vi "ADIS16470 Initialize DMA Odometry.vi"(6 "Encoder R":T1={"DevStatus"={"status"=FALSE, "code"=0, "source"=""}, "EncoderIndex"=enum."Invalid", "CounterIndex"=enum."Invalid", "DistancePerCount"=1.0, "Decoding Type"=enum."4x"}, 7 "Encoder L":T1={"DevStatus"={"status"=FALSE, "code"=0, "source"=""}, "EncoderIndex"=enum."Invalid", "CounterIndex"=enum."Invalid", "DistancePerCount"=1.0, "Decoding Type"=enum."4x"}, 8 "error in":errorcluster, 9 "Calibration Time":T5, 11 "ADIS16470DevRef":T7={"DevStatus"={"status"=FALSE, "code"=0, "source"=""}, "Hardware Config"={"SPI Clock Rate (Hz)"=1000000.0, "IMU SPI Mode (3)"=enum."Mode 3 (Clk Idle High,Sample on Trailing)", "IMU Reset Pin"=enum."SPI Port CS2", "IMU SPI Bus"=enum."SPI On-Board, CS0", "IMU Data Ready Pin"=enum."SPI Port CS1", "Stall Config"={"Pow2BytesPerRead"=255, "StallTicks"=640, "CsToSclkTicks"=5}}, "Calibration Complete"=refnum, "Status FIFO"=refnum, "Last Value Reference"=refnum, "Sychronous Process VI"=refnum, "Cmd FIFO"=refnum, "Source"={"DevStatus"={"status"=FALSE, "code"=0, "source"=""}, "AnalogTriggerMode?"=FALSE, "DigitalMode"={"DIO Channel"=enum."Disabled"}, "AnalogTriggerMode"={"AnalogTriggerIndex"=enum."Trig 0", "OutputType"=enum."InWindow"}}, "Data FIFO"=refnum, "Calibration Time"=enum."1s"}) -> (0 "error out":errorcluster)   [LabVIEW 2019]
uses:
  Typedef/ADIS16470 Device Reference.ctl
  Typedef/ADIS16470 Hardware Configuration.ctl
  <vilib>/Rock Robotics/WPI/SPI/WPI_SPIMode.ctl
  <vilib>/Rock Robotics/SystemInterfaces/DIO/FPGA_DIOChannel.ctl
  <vilib>/Rock Robotics/SystemInterfaces/spilib/spi_bus.ctl
  Typedef/ADIS16470 Status.ctl
  Typedef/ADIS16470 Data.ctl
  Typedef/ADIS16470 Process.ctl
  Typedef/ADIS16470 Command Type.ctl
  <vilib>/Rock Robotics/SystemInterfaces/CounterEncoderSourceConvertion/FPGA_CounterEncoderSourceConvertionLVSourceType.ctl
  <vilib>/Rock Robotics/SystemInterfaces/DIO/FPGA_DIODigitalSourceChannel.ctl
  <vilib>/Rock Robotics/SystemInterfaces/AnalogTrigger/FPGA_AnalogTriggerIndex.ctl
  <vilib>/Rock Robotics/SystemInterfaces/AnalogTrigger/FPGA_AnalogTriggerOutType.ctl
  Typedef/ADIS16470 Calibration Time.ctl
  <vilib>/Rock Robotics/WPI/Encoder/WPI_EncoderDevRef.ctl
  <vilib>/Rock Robotics/SystemInterfaces/Encoder/FPGA_EncoderIdx.ctl
  <vilib>/Rock Robotics/SystemInterfaces/Counter/FPGA_CounterCtrSystemIndex.ctl
  <vilib>/Rock Robotics/WPI/Encoder/WPI_EncoderType.ctl
  <vilib>/Rock Robotics/WPI/SPI/WPI_SPIDevRef.ctl
  Typedef/ADIS16470 Register.ctl
  <vilib>/Rock Robotics/WPI/DMA/WPI_DMARef.ctl
  Typedef/ADIS16470 State Machine.ctl
  <vilib>/Rock Robotics/WPI/DMA/WPI_DMAEncoderOutputType.ctl
  Support Code/Indicator LED - Green.ctl
  Support Code/Indicator LED Indexes.ctl
  <vilib>/Rock Robotics/WPI/Counter/WPI_CounterDigitalInputToDigitalSource.vi
  <vilib>/Rock Robotics/WPI/DMA/WPI_DMAOpenExternal.vi
  <vilib>/Rock Robotics/WPI/DMA/WPI_DMAAddChannelToStream_Encoder.vi
  <vilib>/Rock Robotics/WPI/DMA/WPI_DMAAddChannelToStream_Timestamp.vi
panel:
  out "Array2Prev":u32[](array[numeric])
  out "ArrayPrev":u32[](array[numeric])
  out "Array 2":u32[](array[numeric])
  out "Array":u32[](array[numeric])
  in  "element":T6
  out "Waveform Chart":dbl(graph)
  out "Offset Bias":i16[](array[numeric])
  # "XG_BIAS_LOW"
  # "XG_BIAS_HIGH"
  # "YG_BIAS_LOW"
  # "YG_BIAS_HIGH"
  # "ZG_BIAS_LOW"
  # "ZG_BIAS_HIGH"
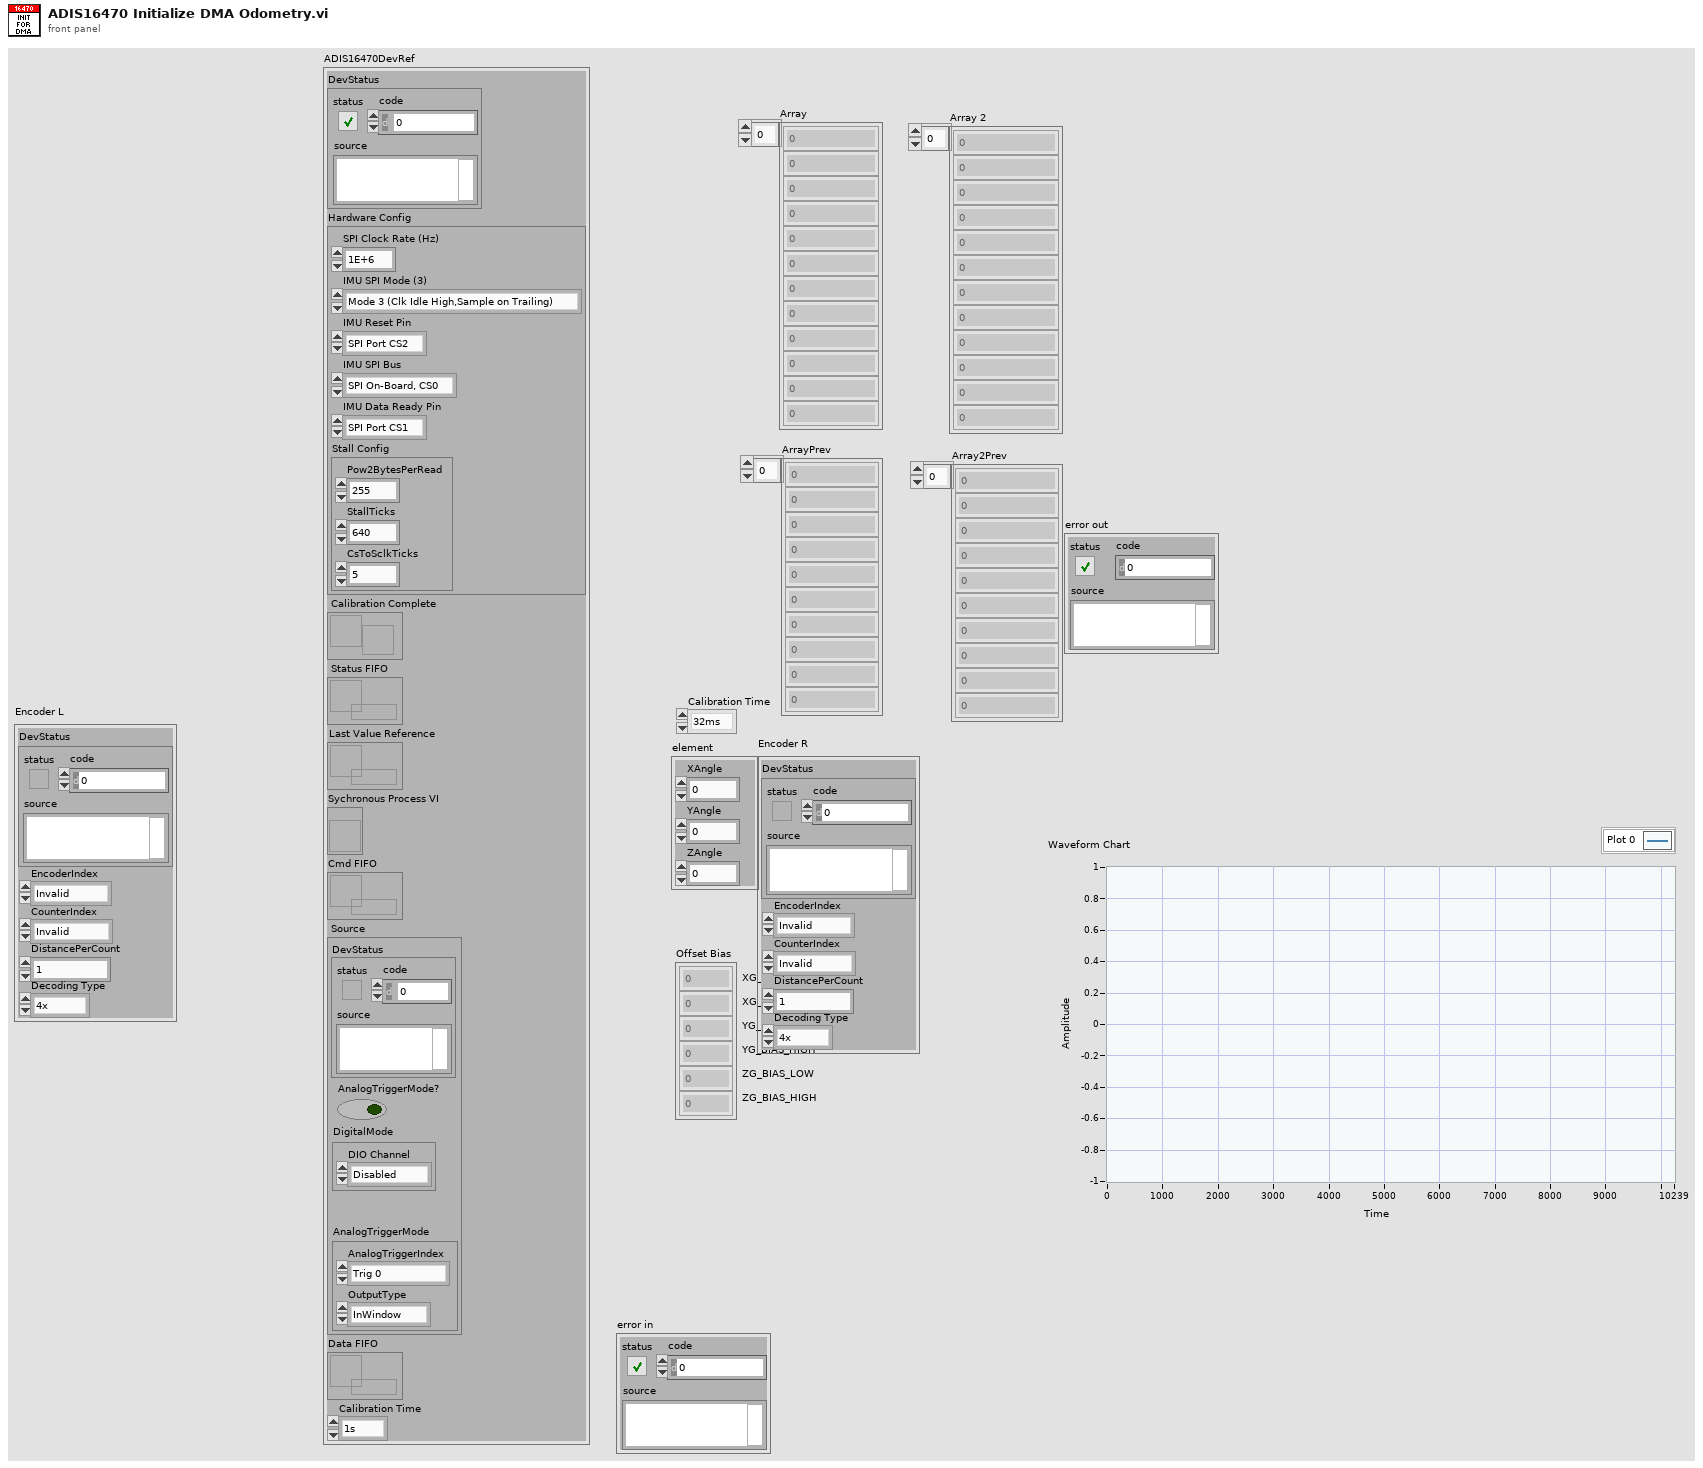
[diagram p1: front panel]
types:
  T1 = typedef "WPI_EncoderDevRef.ctl" = cluster{"DevStatus":errorcluster, "EncoderIndex":T2, "CounterIndex":T3, "DistancePerCount":dbl, "Decoding Type":T4}
  T2 = typedef "FPGA_EncoderIdx.ctl" = enum8{"Enc 0", "Enc 1", "Enc 2", "Enc 3", "Enc 4", "Enc 5", "Enc 6", "Enc 7", "Invalid"}
  T3 = typedef "FPGA_CounterCtrSystemIndex.ctl" = enum8{"Ctr 0", "Ctr 1", "Ctr 2", "Ctr 3", "Ctr 4", "Ctr 5", "Ctr 6", "Ctr 7", "Invalid"}
  T4 = typedef "WPI_EncoderType.ctl" = enum16{"1x", "2x", "4x"}
  T5 = typedef "ADIS16470 Calibration Time.ctl" = enum16{"32ms", "64ms", "128ms", "256ms", "512ms", "1s", "2s", "4s", "8s", "16s", "32s", "64s"}
  T6 = typedef "ADIS16470 Data.ctl" = cluster{"XAngle":dbl, "YAngle":dbl, "ZAngle":dbl}
  T7 = typedef "ADIS16470 Device Reference.ctl" = cluster{"DevStatus":errorcluster, "Hardware Config":T8, "Calibration Complete":refnum<notifier>, "Status FIFO":refnum<k33>, "Last Value Reference":refnum<data-value>, "Sychronous Process VI":T12, "Cmd FIFO":refnum<k33>, "Source":T13, "Data FIFO":refnum<k33>, "Calibration Time":T5}
  T8 = typedef "ADIS16470 Hardware Configuration.ctl" = cluster{"SPI Clock Rate (Hz)":dbl, "IMU SPI Mode (3)":T9, "IMU Reset Pin":T10, "IMU SPI Bus":T11, "IMU Data Ready Pin":T10, "Stall Config":cluster{"Pow2BytesPerRead":u8, "StallTicks":u16, "CsToSclkTicks":u8}}
  T9 = typedef "WPI_SPIMode.ctl" = enum16{"Mode 0 (Clk Idle Low,Sample on Leading)", "Mode 1 (Clk Idle Low,Sample on Trailing)", "Mode 2 (Clk Idle High,Sample on Leading)", "Mode 3 (Clk Idle High,Sample on Trailing)"}
  T10 = typedef "FPGA_DIOChannel.ctl" = enum8{"DIO 0", "DIO 1", "DIO 2", "DIO 3", "DIO 4", "DIO 5", "DIO 6", "DIO 7", "DIO 8", "DIO 9", "DIO MXP 0", "DIO MXP 1", "DIO MXP 2", "DIO MXP 3", "DIO MXP 4", "DIO MXP 5", "DIO MXP 6", "DIO MXP 7", "DIO MXP 8", "DIO MXP 9", "DIO MXP 10", "DIO MXP 11", "DIO MXP 12", "DIO MXP 13", "DIO MXP 14", "DIO MXP 15", "SPI Port CS1", "SPI Port CS2", "SPI Port CS3", "SPI Port MISO", "SPI Port MOSI", "Invalid"}
  T11 = typedef "spi_bus.ctl" = enum16{"SPI On-Board, CS0", "SPI On-Board, CS1", "SPI On-Board, CS2", "SPI On-Board, CS3", "SPI MXP", "Invalid"}
  T12 = typedef "ADIS16470 Process.ctl" = refnum<vi>
  T13 = typedef "FPGA_CounterEncoderSourceConvertionLVSourceType.ctl" = cluster{"DevStatus":errorcluster, "AnalogTriggerMode?":bool, "DigitalMode":cluster{"DIO Channel":T14}, "AnalogTriggerMode":cluster{"AnalogTriggerIndex":T15, "OutputType":T16}}
  T14 = typedef "FPGA_DIODigitalSourceChannel.ctl" = enum8{"DIO 0", "DIO 1", "DIO 2", "DIO 3", "DIO 4", "DIO 5", "DIO 6", "DIO 7", "DIO 8", "DIO 9", "DIO MXP 0", "DIO MXP 1", "DIO MXP 2", "DIO MXP 3", "DIO MXP 4", "DIO MXP 5", "DIO MXP 6", "DIO MXP 7", "DIO MXP 8", "DIO MXP 9", "DIO MXP 10", "DIO MXP 11", "DIO MXP 12", "DIO MXP 13", "DIO MXP 14", "DIO MXP 15", "SPI Port CS1", "SPI Port CS2", "SPI Port CS3", "SPI Port MISO", "SPI Port MOSI", "Disabled"}
  T15 = typedef "FPGA_AnalogTriggerIndex.ctl" = enum8{"Trig 0", "Trig 1", "Trig 2", "Trig 3", "Trig 4", "Trig 5", "Trig 6", "Trig 7", "Invalid"}
  T16 = typedef "FPGA_AnalogTriggerOutType.ctl" = enum16{"InWindow", "TriggerState", "Rising", "Falling"}
  T17 = typedef "ADIS16470 State Machine.ctl" = enum16{"Error", "Reset", "Register DR Source", "Start SPI", "Write Config", "Calibrate", "Write Run Config", "Init Encoder DMA", "Init Auto SPI", "Decode AutoSPI", "Decode Encoder DMA", "Process", "Run Cmds", "Close"}
  T18 = typedef "WPI_SPIDevRef.ctl" = cluster{"DevStatus":errorcluster, "Handle":i32, "SPI Bus":T11}
  T19 = typedef "ADIS16470 Register.ctl" = u8
  T20 = typedef "WPI_DMARef.ctl" = cluster{"DevStatus":errorcluster, "Host Buffer Depth (Samples)":u32}
  T21 = cluster{"SPIDevRef":T18, "Data Counter":u16, "Reset":bool, "Data Ready Source":T13, "Bytes Per Sample":u32, "Data":dbl[], "ADIS16470DevRef":T7, "TimeStampPrev":u32, "Sensor to Robot Rotation":dbl[][], "Data Packet":T19[], "AutoSPI Active?":bool, "Encoder L":T1, "Encoder R":T1, "DMARef":T20, "IMU Raw":cluster{"Theta":dbl[], "Timestamp":u32}[], "Encoder Raw":cluster{"Encoder R":u32, "Encoder L":u32, "Timestamp":u32}[]}
  T22 = typedef "ADIS16470 Status.ctl" = cluster{"Calibrated?":bool, "IMU Detected?":bool}
  T23 = cluster{"DigitalSource":T13, "Edge":enum16{"Rising Edge", "Falling Edge", "Raising & Falling Edge", "Disabled"}}
  T24 = typedef "Indicator LED Indexes.ctl" = enum16{"Code Started", "DS Connected", "Limelight", "Turret Calibrated", "Gyro Calibrated", "USB0 Connected", "USB1 Connected", "FMS Attached"}
  T25 = typedef "Indicator LED - Green.ctl" = u32
  T26 = typedef "ADIS16470 Command Type.ctl" = cluster{"Command":enum16{"None", "Reset", "Set Calibration Period", "Recalibrate", "Recal Complete", "Exit Auto SPI", "Start Auto SPI"}, "Data":u32}
  T27 = typedef "WPI_DigitalOutputDevRef.ctl" = cluster{"DIO Channel":T10, "DevStatus":errorcluster}
  T28 = typedef "WPI_DigitalInputDevRef.ctl" = cluster{"DevStatus":errorcluster, "DIO Channel":T10}
  T29 = typedef "WPI_DMAEncoderOutputType.ctl" = enum16{"Encoder Value", "Timer Value"}
  T30 = cluster{"DigitalSource":T13, "Edge":enum16{"Rising Edge", "Falling Edge", "Raising & Falling Edge", "Disabled"}}[]
  T31 = cluster{"Pow2BytesPerRead":u8, "StallTicks":u16, "CsToSclkTicks":u8}
  T32 = cluster{"Encoder R":i32, "Encoder L":i32, "Timestamp":u32}[]
  T33 = cluster{"Encoder R":u32, "Encoder L":u32, "Timestamp":u32}[]
  T34 = enum16{"None", "Reset", "Set Calibration Period", "Recalibrate", "Recal Complete", "Exit Auto SPI", "Start Auto SPI"}
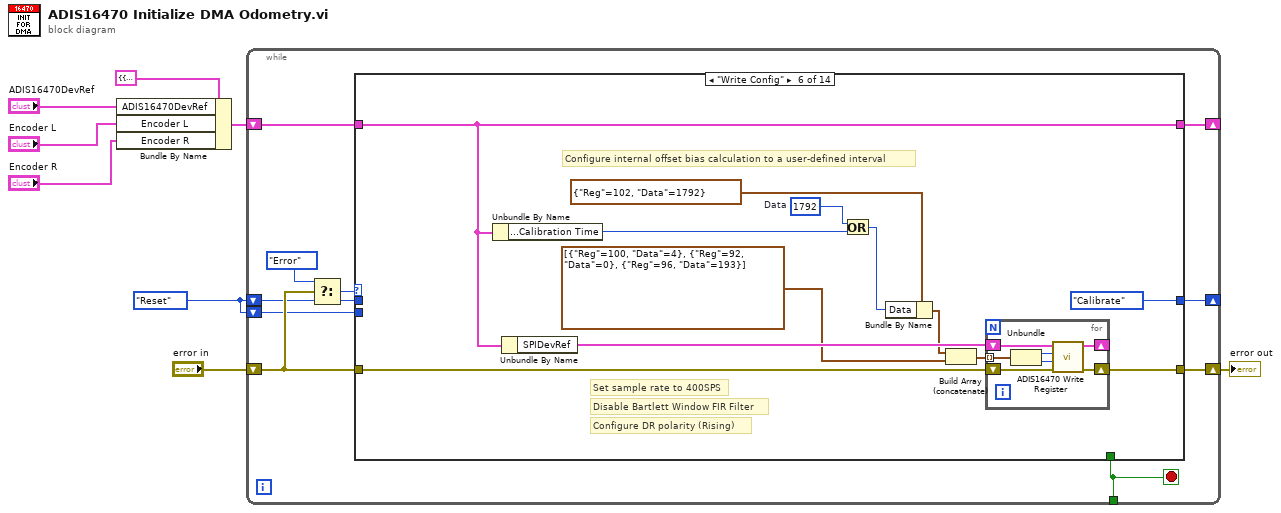
[diagram p0: block diagram]
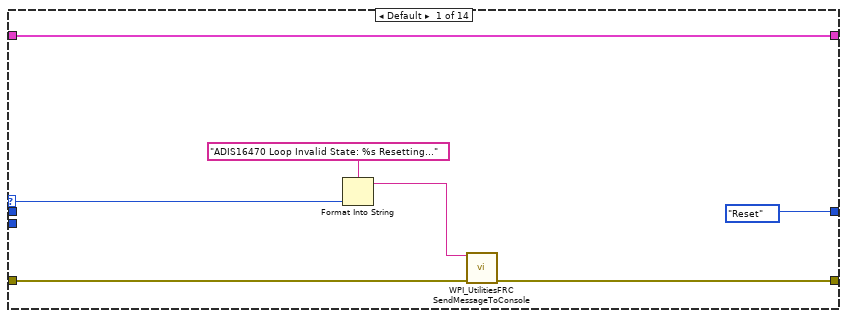
[diagram p2: hidden frame]
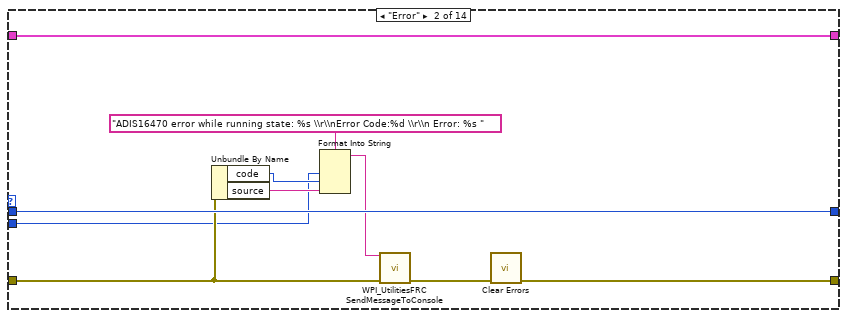
[diagram p3: hidden frame]
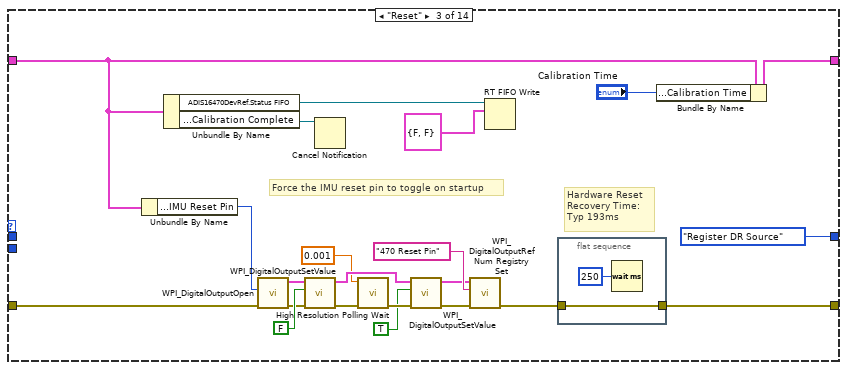
[diagram p4: hidden frame]
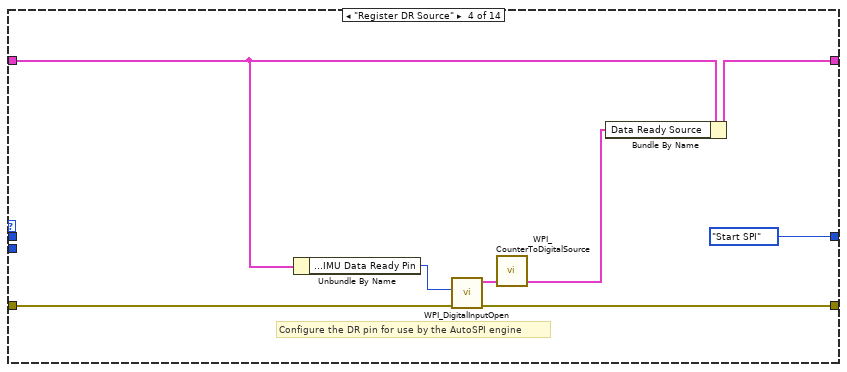
[diagram p5: hidden frame]
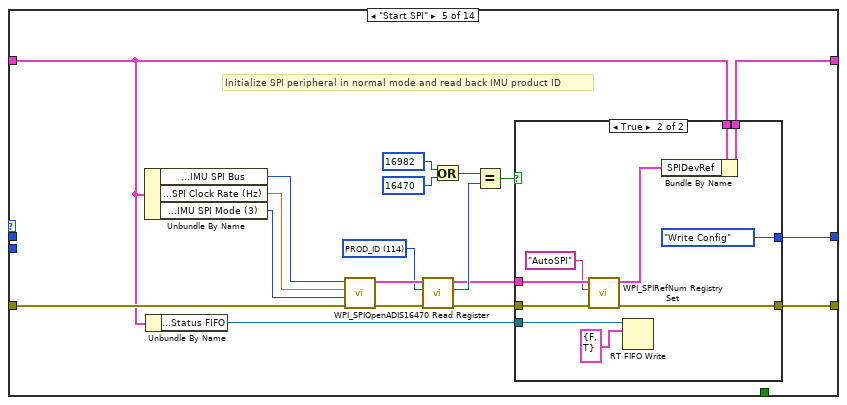
[diagram p6: hidden frame]
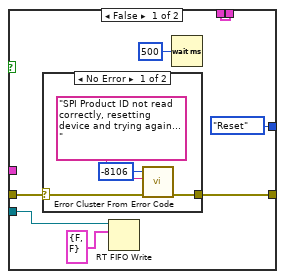
[diagram p7: hidden frame]
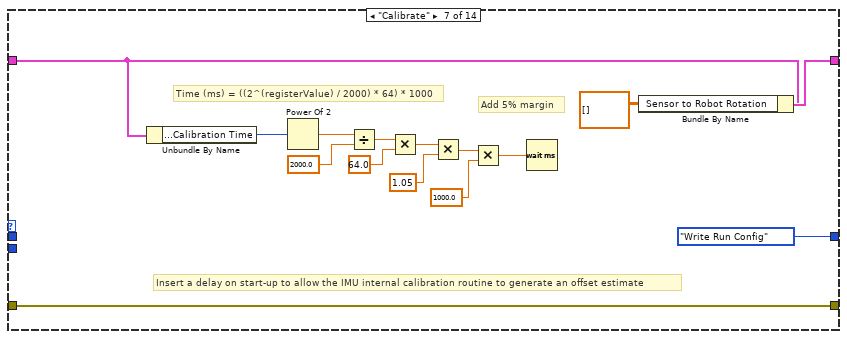
[diagram p9: hidden frame]
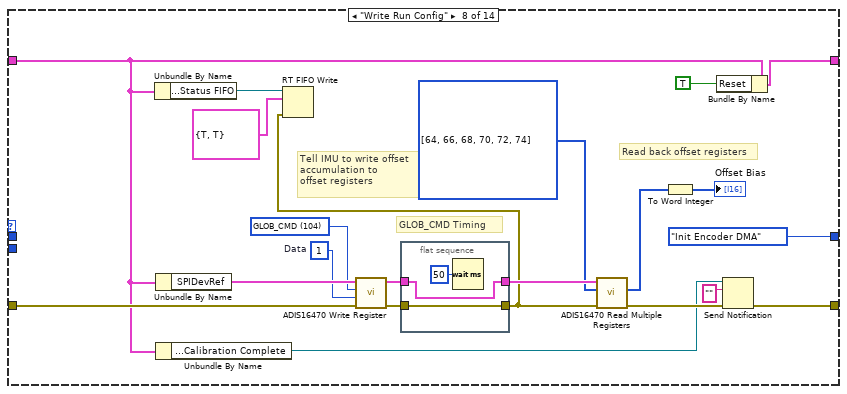
[diagram p10: hidden frame]
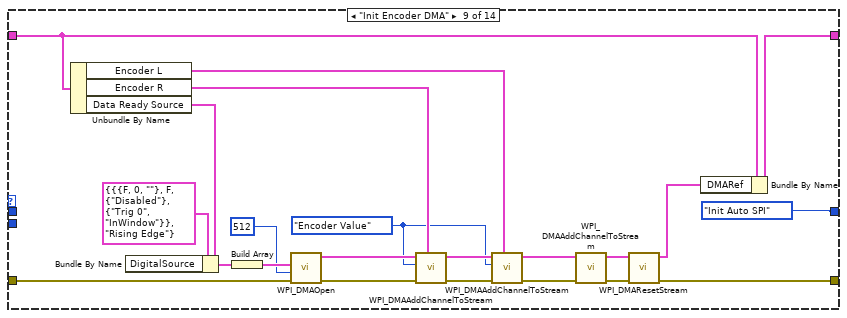
[diagram p11: hidden frame]
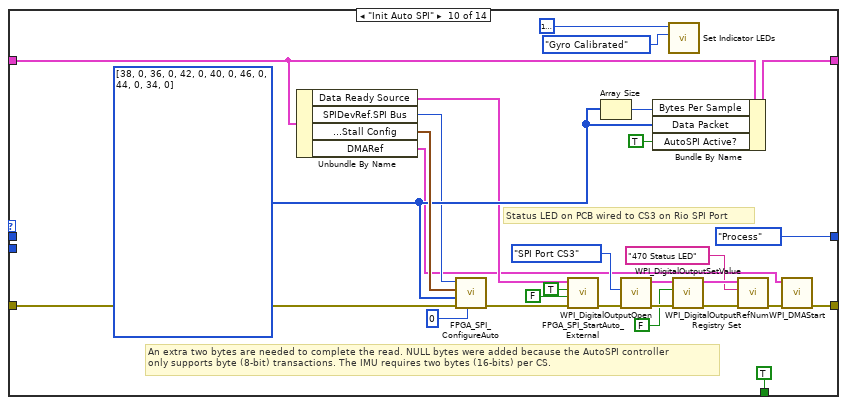
[diagram p12: hidden frame]
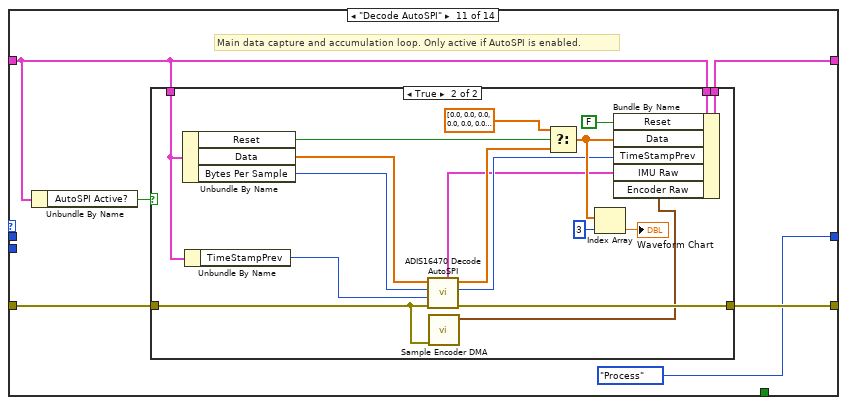
[diagram p13: hidden frame]
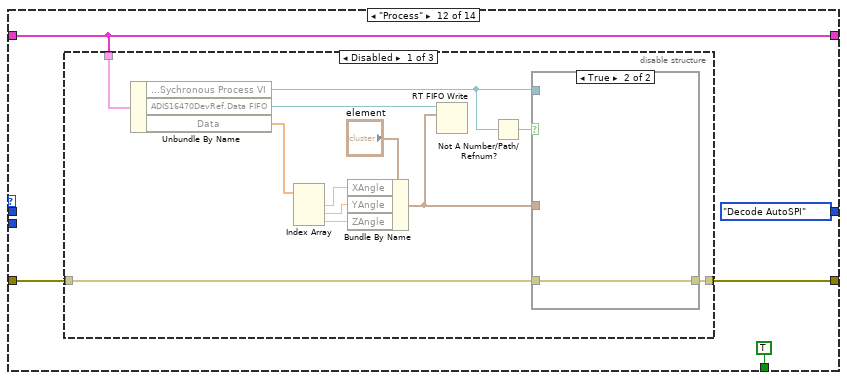
[diagram p15: hidden frame]
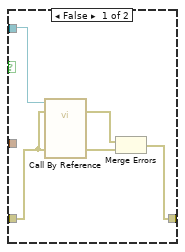
[diagram p16: hidden frame]
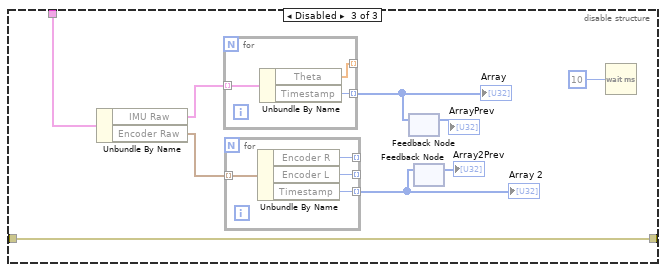
[diagram p18: hidden frame]
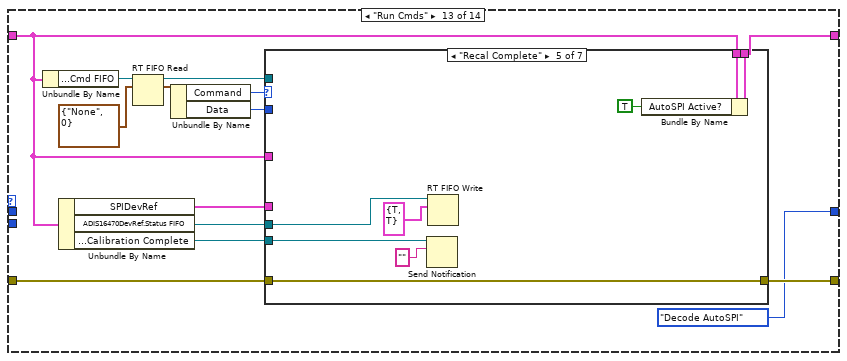
[diagram p19: hidden frame]
diagram:
  w4 = ADIS16470_State_Machine."Reset" ("ADIS16470 State Machine")
  n1 = Bundle By Name(cluster=T21 {"SPIDevRef"={"DevStatus"={"status"=FALSE, "code"=0, "source"=""}, "Handle"=0, "SPI Bus"=enum."SPI On-Board, CS0"}, "Data Counter"=0, "Reset"=FALSE, "Data Ready Source"={"DevStatus"={"status"=FALSE, "code"=0, "source"=""}, "AnalogTriggerMode?"=FALSE, "DigitalMode"={"DIO Channel"=enum."DIO 1"}, "AnalogTriggerMode"={"AnalogTriggerIndex"=enum."Trig 0", "OutputType"=enum."InWindow"}}, "Bytes Per Sample"=0, "Data"=[0.0, 0.0, 0.0, 0.0, 0.0, 0.0, 0.0, 0.0], "ADIS16470DevRef"={"DevStatus"={"status"=FALSE, "code"=0, "source"=""}, "Hardware Config"={"SPI Clock Rate (Hz)"=1000000.0, "IMU SPI Mode (3)"=enum."Mode 3 (Clk Idle High,Sample on Trailing)", "IMU Reset Pin"=enum."SPI Port CS2", "IMU SPI Bus"=enum."SPI On-Board, CS0", "IMU Data Ready Pin"=enum."SPI Port CS1", "Stall Config"={"Pow2BytesPerRead"=255, "StallTicks"=640, "CsToSclkTicks"=5}}, "Calibration Complete"=refnum, "Status FIFO"=refnum, "Last Value Reference"=refnum, "Sychronous Process VI"=refnum, "Cmd FIFO"=refnum, "Source"={"DevStatus"={"status"=FALSE, "code"=0, "source"=""}, "AnalogTriggerMode?"=FALSE, "DigitalMode"={"DIO Channel"=enum."Disabled"}, "AnalogTriggerMode"={"AnalogTriggerIndex"=enum."Trig 0", "OutputType"=enum."InWindow"}}, "Data FIFO"=refnum, "Calibration Time"=enum."1s"}, "TimeStampPrev"=0, "Sensor to Robot Rotation"=[], "Data Packet"=[38, 0, 36, 0, 42, 0, 40, 0, 46, 0, 44, 0, 114, 0], "AutoSPI Active?"=TRUE, "Encoder L"={"DevStatus"={"status"=FALSE, "code"=0, "source"=""}, "EncoderIndex"=enum."Invalid", "CounterIndex"=enum."Invalid", "DistancePerCount"=1.0, "Decoding Type"=enum."4x"}, "Encoder R"={"DevStatus"={"status"=FALSE, "code"=0, "source"=""}, "EncoderIndex"=enum."Invalid", "CounterIndex"=enum."Invalid", "DistancePerCount"=1.0, "Decoding Type"=enum."4x"}, "DMARef"={"DevStatus"={"status"=FALSE, "code"=0, "source"=""}, "Host Buffer Depth (Samples)"=0}, "IMU Raw"=[], "Encoder Raw"=[]}, "ADIS16470DevRef"="ADIS16470DevRef", "Encoder L"="Encoder L", "Encoder R"="Encoder R") -> (w7:T21)
  n2 = while {
    shift-right: [w15] -> _
    shift-left: w4 -> [w12]
    shift-right: [w17] -> _
    shift-left: w7 -> [w18]
    shift-right: [w16] -> w1
    shift-left: "error in" -> [w14]
    shift-left: w4 -> [w11]
    tunnel: [w9] -> _
    stop <- w9 stop-if-true
    n3 = Select(t=ADIS16470_State_Machine."Error" ("ADIS16470 State Machine"), s=w14, f=w12) -> (s? t:f=w13:T17)
    n4 = case shown="\"Write Config\"" w13 {
      selector: w13 -> [w24 _ _ _ _ _ _ _ _ _ _ _ _ _]
      tunnel: w18 -> [w25 w35 w39 w64 w69 w111 w139 w149 w188 w209 w219 w247 w284 w410]
      tunnel: [w25 w35 w38 w67 w77 w111 w141 w156 w174 w208 w222 w247 w291 w410] -> w17
      tunnel: w14 -> [w23 w31 w55 w66 w83 w119 w140 w162 w181 w216 w221 w246 w293 w409]
      tunnel: [w22 w32 w54 w61 w76 w118 w140 w151 w169 w193 w220 w245 w292 w409] -> w16
      tunnel: [ADIS16470_State_Machine."Reset" ("ADIS16470 State Machine") w34 ADIS16470_State_Machine."Register DR Source" ("ADIS16470 State Machine") ADIS16470_State_Machine."Start SPI" ("ADIS16470 State Machine") w78 ADIS16470_State_Machine."Calibrate" ("ADIS16470 State Machine") ADIS16470_State_Machine."Write Run Config" ("ADIS16470 State Machine") ADIS16470_State_Machine."Init Encoder DMA" ("ADIS16470 State Machine") ADIS16470_State_Machine."Init Auto SPI" ("ADIS16470 State Machine") ADIS16470_State_Machine."Process" ("ADIS16470 State Machine") ADIS16470_State_Machine."Process" ("ADIS16470 State Machine") ADIS16470_State_Machine."Decode AutoSPI" ("ADIS16470 State Machine") ADIS16470_State_Machine."Decode AutoSPI" ("ADIS16470 State Machine") ADIS16470_State_Machine."Reset" ("ADIS16470 State Machine")] -> w15
      tunnel: w12 -> [_ w34 _ _ _ _ _ _ _ _ _ _ _ _]
      tunnel: w11 -> [_ w26 _ _ _ _ _ _ _ _ _ _ _ _]
      tunnel: [_ _ _ _ _ _ _ _ _ TRUE _ TRUE _ TRUE] -> w9
      frame Default {
        n5 = Format Into String(format string="ADIS16470 Loop Invalid State: %s Resetting...", w24) -> (resulting string=w21:string)  [unwired: 2 in, 1 out]
        n6 = call <vilib>:"WPI_UtilitiesFRC SendMessageToConsole.vi"("Message"=w21, "error in (no error)"=w23) -> ("error out"=w22:errorcluster)  [unwired: 13 in]
      }
      frame "Error" {
        n7 = Unbundle By Name(w31) -> ("code"=w28:i32, "source"=w27:string)
        n8 = Format Into String(format string="ADIS16470 error while running state: %s \\r\\nError Code:%d \\r\\n Error: %s ", w26, w28, w27) -> (resulting string=w30:string)  [unwired: 2 in, 1 out]
        n9 = call <vilib>:"WPI_UtilitiesFRC SendMessageToConsole.vi"("Message"=w30, "error in (no error)"=w31) -> ("error out"=w33:errorcluster)  [unwired: 13 in]
        n10 = call <vilib>:"Clear Errors.vi"("error in (no error)"=w33) -> ("error out"=w32:errorcluster)  [unwired: 5 in, 1 out]
      }
      frame "Reset" {
        # "Hardware Reset Recovery Time: Typ 193ms"
        # "Force the IMU reset pin to toggle on startup"
        n11 = Unbundle By Name(w39) -> ("ADIS16470DevRef.Hardware Config.IMU Reset Pin"=w56:T10)
        n12 = Unbundle By Name(w39) -> ("ADIS16470DevRef.Status FIFO"=w52:refnum<k33>, "ADIS16470DevRef.Calibration Complete"=w53:refnum<notifier>)
        n13 = call <vilib>:"WPI_DigitalOutputOpen.vi"("error in (no error)"=w55, "DIO Channel"=w56) -> ("error out"=w49:errorcluster, "DigitalOutputDevRef"=w57:T27)  [unwired: 8 in]
        n14 = call <vilib>:"WPI_DigitalOutputSetValue.vi"("error in (no error)"=w49, "Value"=FALSE, "DigitalOutputDevRef"=w57) -> ("error out"=w46:errorcluster, "DigitalOutputDevRef"=w44:T27)  [unwired: 7 in]
        n15 = Cancel Notification(0:w53) -> ()  [unwired: 1 in, 3 out]
        n16 = call <vilib>:"High Resolution Polling Wait.vi"("error in (no error)"=w46, "seconds to wait"=0.001) -> ("error out"=w45:errorcluster)  [unwired: 9 in]
        n17 = call <vilib>:"WPI_DigitalOutputSetValue.vi"("error in (no error)"=w45, "Value"=TRUE, "DigitalOutputDevRef"=w44) -> ("error out"=w41:errorcluster, "DigitalOutputDevRef"=w42:T27)  [unwired: 7 in]
        n18 = call <vilib>:"WPI_DigitalOutputRefNum Registry Set.vi"("error in (no error)"=w41, "refnum name"="470 Reset Pin", "DigitalOutputDevRef"=w42) -> ("error out"=w47:errorcluster)  [unwired: 7 in, 1 out]
        n19 = RT FIFO Write(0:w52, 1:T22 {"Calibrated?"=FALSE, "IMU Detected?"=FALSE} ("element")) -> ()  [unwired: 3 in, 4 out]
        n20 = flat-sequence {
          tunnel: [w59] -> w54
          tunnel: w47 -> [w59]
          frame #0 {
            n21 = Wait (ms)(milliseconds to wait=u32 250) -> ()  [unwired: 1 out]
          }
        }
        n22 = Bundle By Name(cluster=w39, "ADIS16470DevRef.Calibration Time"="Calibration Time") -> (w38:T21)
      }
      frame "Register DR Source" {
        # "Configure the DR pin for use by the AutoSPI engine"
        n23 = Unbundle By Name(w64) -> ("ADIS16470DevRef.Hardware Config.IMU Data Ready Pin"=w63:T10)
        n24 = call <vilib>:"WPI_DigitalInputOpen.vi"("error in (no error)"=w66, "DIO Channel"=w63) -> ("error out"=w61:errorcluster, "DigitalInputDevRef"=w65:T28)  [unwired: 8 in]
        n25 = call-poly <vilib>:"WPI_CounterToDigitalSource.vi"("DigitalInputDevRef"=w65) -> ("Digital Source"=w62:T13)  [unwired: 6 in]
        n26 = Bundle By Name(cluster=w64, "Data Ready Source"=w62) -> (w67:T21)
      }
      frame "Start SPI" {
        w71 = T19 114 items=["Reserved1"=0, "DIAG_STAT"=2, "X_GYRO_LOW"=4, "X_GYRO_OUT"=6, "Y_GYRO_LOW"=8, "Y_GYRO_OUT"=10, "Z_GYRO_LOW"=12, "Z_GYRO_OUT"=14, "X_ACCL_LOW"=16, "X_ACCL_OUT"=18, "Y_ACCL_LOW"=20, "Y_ACCL_OUT"=22, "Z_ACCL_LOW"=24, "Z_ACCL_OUT"=26, "TEMP_OUT"=28, "TIME_STAMP"=30, "Reseved2"=32, "DATA_CNTR"=34, "X_DELTANG_LOW"=36, "X_DELTANG_OUT"=38, "Y_DELTANG_LOW"=40, "Y_DELTANG_OUT"=42, "Z_DELTANG_LOW"=44, "Z_DELTANG_OUT"=46, "X_DELTVEL_LOW"=48, "X_DELTVEL_OUT"=50, "Y_DELTVEL_LOW"=52, "Y_DELTVEL_OUT"=54, "Z_DELTVEL_LOW"=56, "Z_DELTVEL_OUT"=58, "Reserved3"=60, "Reserved4"=62, "XG_BIAS_LOW"=64, "XG_BIAS_HIGH"=66, "YG_BIAS_LOW"=68, "YG_BIAS_OUT"=70, "ZG_BIAS_LOW"=72, "ZG_BIAS_OUT"=74, "XA_BIAS_LOW"=76, "XA_BIAS_HIGH"=78, "YA_BIAS_LOW"=80, "YA_BIAS_OUT"=82, "ZA_BIAS_LOW"=84, "ZA_BIAS_OUT"=86, "Reserved5"=88, "Reserved6"=90, "FILT_CTRL"=92, "Reserved5"=94, "MSC_CTRL"=96, "UP_SCALE"=98, "DEC_RATE"=100, "NULL_CNFG"=102, "GLOB_CMD"=104, "Reserved6"=106, "FIRM_REV"=108, "FIRM_DM"=110, "FIRM_Y"=112, "PROD_ID"=114, "SERIAL_NUM"=116, "USER_SCR1"=118, "USER_SCR2"=120, "USER_SCR3"=122, "FLSHCNT_LOW"=124, "FLSHCNT_HIGH"=126] ("ADIS16448 Register")
        # "Initialize SPI peripheral in normal mode and read back IMU product ID"
        n27 = Unbundle By Name(w69) -> ("ADIS16470DevRef.Hardware Config.IMU SPI Bus"=w79:T11, "ADIS16470DevRef.Hardware Config.SPI Clock Rate (Hz)"=w80:dbl, "ADIS16470DevRef.Hardware Config.IMU SPI Mode (3)"=w81:T9)
        n28 = Unbundle By Name(w69) -> ("ADIS16470DevRef.Status FIFO"=w68:refnum<k33>)
        n29 = call <vilib>:"WPI_SPIOpen.vi"("error in"=w83, "Mode (3)"=w81, "Clock Rate (Hz)"=w80, "SPI Bus"=w79) -> ("error out"=w73:errorcluster, "SPIDevRef"=w72:T18)  [unwired: 6 in]
        n30 = call "ADIS16470 Read Register.vi"("error in (no error)"=w73, "ADIS16470 Register"=w71, "SPIDevRef in"=w72) -> ("error out"=w74:errorcluster, "Register Value"=w75:u16, "SPIDevRef out"=w70:T18)  [unwired: 6 in]
        n31 = Or(x=u16 16982 ("y"), y=u16 16470) -> (x .or. y?=w84:u16)
        n32 = Equal?(x=w84, y=w75) -> (x = y?=w82:bool)
        n33 = case shown="True" w82 {
          tunnel: [ADIS16470_State_Machine."Reset" ("ADIS16470 State Machine") ADIS16470_State_Machine."Write Config" ("ADIS16470 State Machine")] -> w78
          tunnel: w69 -> [w93 w108]
          tunnel: [w93 w107] -> w77
          tunnel: [w92 w103] -> w76
          tunnel: w74 -> [w91 w106]
          tunnel: w70 -> [_ w105]
          tunnel: w68 -> [w89 w101]
          frame False {
            n34 = case shown="No Error" w91 {
              selector: w91 -> [w96 w98]
              tunnel: [w97 w98] -> w92
              frame No Error {
                n35 = call <vilib>:"Error Cluster From Error Code.vi"("error in (no error)"=w96, "error message (\"\")"="SPI Product ID not read correctly, resetting device and trying again..." ("error message (\"\")"), "error code (0)"=-8106) -> ("error out"=w97:errorcluster)  [unwired: 6 in]
              }
              frame Error {
              }
            }
            n36 = RT FIFO Write(0:w89, 1:T22 {"Calibrated?"=FALSE, "IMU Detected?"=FALSE} ("element")) -> ()  [unwired: 3 in, 4 out]
            n37 = Wait (ms)(milliseconds to wait=u32 500) -> ()  [unwired: 1 out]
          }
          frame True {
            n38 = call <vilib>:"WPI_SPIRefNum Registry Set.vi"("error in (no error)"=w106, "refnum name"="AutoSPI", "SPIDevRef"=w105) -> ("error out"=w103:errorcluster, "SPIDevRef"=w104:T18)  [unwired: 7 in]
            n39 = RT FIFO Write(0:w101, 1:T22 {"Calibrated?"=FALSE, "IMU Detected?"=TRUE} ("element")) -> ()  [unwired: 3 in, 4 out]
            n40 = Bundle By Name(cluster=w108, "SPIDevRef"=w104) -> (w107:T21)
          }
        }
      }
      frame "Write Config" {
        w113 = 1792  # Data
        # "Set sample rate to 400SPS"
        # "Configure internal offset bias calculation to a user-defined interval"
        # "Configure DR polarity (Rising)"
        # "Disable Bartlett Window FIR Filter"
        n41 = Unbundle By Name(w111) -> ("ADIS16470DevRef.Calibration Time"=w110:T5)
        n42 = Unbundle By Name(w111) -> ("SPIDevRef"=w120:T18)
        n43 = Or(x=w113, y=w110) -> (x .or. y?=w112:i32)
        n44 = Bundle By Name(cluster=cluster{"Reg":T19, "Data":i32} {"Reg"=102, "Data"=1792}, "Data"=w112) -> (w114:cluster{"Reg":T19, "Data":i32})
        n45 = Build Array (concatenate)(w114, cluster{"Reg":T19, "Data":u16}[] [{"Reg"=100, "Data"=4}, {"Reg"=92, "Data"=0}, {"Reg"=96, "Data"=193}]) -> (w115:cluster{"Reg":T19, "Data":i32}[])
        n46 = for {
          tunnel: w115 -> [w127] mode=indexing
          shift-right: [w123] -> w118
          shift-left: w119 -> [w122]
          shift-right: [w121] -> _
          shift-left: w120 -> [w124]
          n47 = Unbundle(w127) -> ("Reg"=w126:T19, "Data"=w125:i32)
          n48 = call "ADIS16470 Write Register.vi"("error in (no error)"=w122, "Data"=w125, "Register"=w126, "SPIDevRef in"=w124) -> ("error out"=w123:errorcluster, "SPIDevRef out"=w121:T18)  [unwired: 6 in]
        }
      }
      frame "Calibrate" {
        # "Insert a delay on start-up to allow the IMU internal calibration routine to generate an offset estimate"
        # "Add 5% margin"
        # "Time (ms) = ((2^(registerValue) / 2000) * 64) * 1000"
        n49 = Unbundle By Name(w139) -> ("ADIS16470DevRef.Calibration Time"=w138:T5)
        n50 = Power Of 2(x=w138) -> (2^x=w137:dbl)
        n51 = Divide(x=w137, y=2000.0) -> (x/y=w135:dbl)
        n52 = Multiply(x=w135, y=64.0) -> (x*y=w133:dbl)
        n53 = Multiply(x=w133, y=1.05) -> (x*y=w131:dbl)
        n54 = Multiply(x=w131, y=1000.0) -> (x*y=w129:dbl)
        n55 = Wait (ms)(milliseconds to wait=w129) -> ()  [unwired: 1 out]
        n56 = Bundle By Name(cluster=w139, "Sensor to Robot Rotation"=dbl[][] []) -> (w141:T21)
      }
      frame "Write Run Config" {
        w146 = T19 104 items=["Reserved1"=0, "DIAG_STAT"=2, "X_GYRO_LOW"=4, "X_GYRO_OUT"=6, "Y_GYRO_LOW"=8, "Y_GYRO_OUT"=10, "Z_GYRO_LOW"=12, "Z_GYRO_OUT"=14, "X_ACCL_LOW"=16, "X_ACCL_OUT"=18, "Y_ACCL_LOW"=20, "Y_ACCL_OUT"=22, "Z_ACCL_LOW"=24, "Z_ACCL_OUT"=26, "TEMP_OUT"=28, "TIME_STAMP"=30, "Reseved2"=32, "DATA_CNTR"=34, "X_DELTANG_LOW"=36, "X_DELTANG_OUT"=38, "Y_DELTANG_LOW"=40, "Y_DELTANG_OUT"=42, "Z_DELTANG_LOW"=44, "Z_DELTANG_OUT"=46, "X_DELTVEL_LOW"=48, "X_DELTVEL_OUT"=50, "Y_DELTVEL_LOW"=52, "Y_DELTVEL_OUT"=54, "Z_DELTVEL_LOW"=56, "Z_DELTVEL_OUT"=58, "Reserved3"=60, "Reserved4"=62, "XG_BIAS_LOW"=64, "XG_BIAS_HIGH"=66, "YG_BIAS_LOW"=68, "YG_BIAS_OUT"=70, "ZG_BIAS_LOW"=72, "ZG_BIAS_OUT"=74, "XA_BIAS_LOW"=76, "XA_BIAS_HIGH"=78, "YA_BIAS_LOW"=80, "YA_BIAS_OUT"=82, "ZA_BIAS_LOW"=84, "ZA_BIAS_OUT"=86, "Reserved5"=88, "Reserved6"=90, "FILT_CTRL"=92, "Reserved5"=94, "MSC_CTRL"=96, "UP_SCALE"=98, "DEC_RATE"=100, "NULL_CNFG"=102, "GLOB_CMD"=104, "Reserved6"=106, "FIRM_REV"=108, "FIRM_DM"=110, "FIRM_Y"=112, "PROD_ID"=114, "SERIAL_NUM"=116, "USER_SCR1"=118, "USER_SCR2"=120, "USER_SCR3"=122, "FLSHCNT_LOW"=124, "FLSHCNT_HIGH"=126] ("Register")
        w161 = u16 1  # Data
        w157 = T19[] [64, 66, 68, 70, 72, 74] items=["Reserved1"=0, "DIAG_STAT"=2, "X_GYRO_LOW"=4, "X_GYRO_OUT"=6, "Y_GYRO_LOW"=8, "Y_GYRO_OUT"=10, "Z_GYRO_LOW"=12, "Z_GYRO_OUT"=14, "X_ACCL_LOW"=16, "X_ACCL_OUT"=18, "Y_ACCL_LOW"=20, "Y_ACCL_OUT"=22, "Z_ACCL_LOW"=24, "Z_ACCL_OUT"=26, "TEMP_OUT"=28, "TIME_STAMP"=30, "Reseved2"=32, "DATA_CNTR"=34, "X_DELTANG_LOW"=36, "X_DELTANG_OUT"=38, "Y_DELTANG_LOW"=40, "Y_DELTANG_OUT"=42, "Z_DELTANG_LOW"=44, "Z_DELTANG_OUT"=46, "X_DELTVEL_LOW"=48, "X_DELTVEL_OUT"=50, "Y_DELTVEL_LOW"=52, "Y_DELTVEL_OUT"=54, "Z_DELTVEL_LOW"=56, "Z_DELTVEL_OUT"=58, "Reserved3"=60, "Reserved4"=62, "XG_BIAS_LOW"=64, "XG_BIAS_HIGH"=66, "YG_BIAS_LOW"=68, "YG_BIAS_HIGH"=70, "ZG_BIAS_LOW"=72, "ZG_BIAS_HIGH"=74, "XA_BIAS_LOW"=76, "XA_BIAS_HIGH"=78, "YA_BIAS_LOW"=80, "YA_BIAS_HIGH"=82, "ZA_BIAS_LOW"=84, "ZA_BIAS_HIGH"=86, "Reserved5"=88, "Reserved6"=90, "FILT_CTRL"=92, "Reserved5"=94, "MSC_CTRL"=96, "UP_SCALE"=98, "DEC_RATE"=100, "NULL_CNFG"=102, "GLOB_CMD"=104, "Reserved6"=106, "FIRM_REV"=108, "FIRM_DM"=110, "FIRM_Y"=112, "PROD_ID"=114, "SERIAL_NUM"=116, "USER_SCR1"=118, "USER_SCR2"=120, "USER_SCR3"=122, "FLSHCNT_LOW"=124, "FLSHCNT_HIGH"=126] ("Registers")
        # "Tell IMU to write offset \naccumulation to \noffset registers"
        # "GLOB_CMD Timing"
        # "Read back offset registers"
        n57 = Unbundle By Name(w149) -> ("ADIS16470DevRef.Status FIFO"=w148:refnum<k33>)
        n58 = Unbundle By Name(w149) -> ("SPIDevRef"=w163:T18)
        n59 = Unbundle By Name(w149) -> ("ADIS16470DevRef.Calibration Complete"=w152:refnum<notifier>)
        n60 = RT FIFO Write(0:w148, 1:T22 {"Calibrated?"=TRUE, "IMU Detected?"=TRUE} ("element"), 3:w145) -> ()  [unwired: 2 in, 4 out]
        n61 = call "ADIS16470 Write Register.vi"("error in (no error)"=w162, "Data"=w161, "Register"=w146, "SPIDevRef in"=w163) -> ("error out"=w160:errorcluster, "SPIDevRef out"=w159:T18)  [unwired: 6 in]
        n62 = flat-sequence {
          tunnel: w160 -> [w166]
          tunnel: [w166] -> w145
          tunnel: w159 -> [w164]
          tunnel: [w164] -> w158
          frame #0 {
            n63 = Wait (ms)(milliseconds to wait=u32 50) -> ()  [unwired: 1 out]
          }
        }
        n64 = call "ADIS16470 Read Multiple Registers.vi"("error in (no error)"=w145, "Registers"=w157, "SPIDevRefIn"=w158) -> ("error out"=w153:errorcluster, "Values"=w144:u16[])  [unwired: 6 in, 1 out]
        n65 = To Word Integer(number=w144) -> (16bit integer=→"Offset Bias":i16[])
        n66 = Bundle By Name(cluster=w149, "Reset"=TRUE ("First Run")) -> (w156:T21)
        n67 = Send Notification(notification="", notifier=w152, error in (no error)=w153) -> (error out=w151:errorcluster)  [unwired: 1 out]
      }
      frame "Init Encoder DMA" {
        w171 = WPI_DMAEncoderOutputType."Encoder Value" ("Encoder Output Type")
        n68 = Unbundle By Name(w188) -> ("Encoder L"=w173:T1, "Encoder R"=w172:T1, "Data Ready Source"=w184:T13)
        n69 = Bundle By Name(cluster=T23 {"DigitalSource"={"DevStatus"={"status"=FALSE, "code"=0, "source"=""}, "AnalogTriggerMode?"=FALSE, "DigitalMode"={"DIO Channel"=enum."Disabled"}, "AnalogTriggerMode"={"AnalogTriggerIndex"=enum."Trig 0", "OutputType"=enum."InWindow"}}, "Edge"=enum."Rising Edge"} ("ExternalSampleClock"), "DigitalSource"=w184) -> (w183:T23)
        n70 = Build Array(w183) -> (w182:T30)
        n71 = call-poly <vilib>:"WPI_DMAOpen.vi"("error in (no error)"=w181, "Host Buffer Depth (Samples)"=u32 512, "ExternalSampleClocks"=w182) -> ("error out"=w180:errorcluster, "DMARef"=w187:T20)  [unwired: 7 in]
        n72 = call-poly <vilib>:"WPI_DMAAddChannelToStream.vi"("EncoderDevRef"=w172, "error in (no error)"=w180, "Encoder Output Type"=w171, "DMARef"=w187) -> ("error out"=w179:errorcluster, "DMARef"=w186:T20)  [unwired: 6 in]
        n73 = call-poly <vilib>:"WPI_DMAAddChannelToStream.vi"("EncoderDevRef"=w173, "error in (no error)"=w179, "Encoder Output Type"=w171, "DMARef"=w186) -> ("error out"=w175:errorcluster, "DMARef"=w177:T20)  [unwired: 6 in]
        n74 = call-poly <vilib>:"WPI_DMAAddChannelToStream.vi"("error in (no error)"=w175, "DMARef"=w177) -> ("error out"=w176:errorcluster, "DMARef"=w168:T20)  [unwired: 8 in]
        n75 = call <vilib>:"WPI_DMAResetStream.vi"("error in (no error)"=w176, "DMARef"=w168) -> ("error out"=w169:errorcluster, "DMARef"=w167:T20)  [unwired: 8 in]
        n76 = Bundle By Name(cluster=w188, "DMARef"=w167) -> (w174:T21)
      }
      frame "Init Auto SPI" {
        w198 = T19[] [38, 0, 36, 0, 42, 0, 40, 0, 46, 0, 44, 0, 34, 0] items=["NULL"=0, "DIAG_STAT"=2, "X_GYRO_LOW"=4, "X_GYRO_OUT"=6, "Y_GYRO_LOW"=8, "Y_GYRO_OUT"=10, "Z_GYRO_LOW"=12, "Z_GYRO_OUT"=14, "X_ACCL_LOW"=16, "X_ACCL_OUT"=18, "Y_ACCL_LOW"=20, "Y_ACCL_OUT"=22, "Z_ACCL_LOW"=24, "Z_ACCL_OUT"=26, "TEMP_OUT"=28, "TIME_STAMP"=30, "Reseved2"=32, "DATA_CNTR"=34, "X_DELTANG_LOW"=36, "X_DELTANG_OUT"=38, "Y_DELTANG_LOW"=40, "Y_DELTANG_OUT"=42, "Z_DELTANG_LOW"=44, "Z_DELTANG_OUT"=46, "X_DELTVEL_LOW"=48, "X_DELTVEL_OUT"=50, "Y_DELTVEL_LOW"=52, "Y_DELTVEL_OUT"=54, "Z_DELTVEL_LOW"=56, "Z_DELTVEL_OUT"=58, "Reserved3"=60, "Reserved4"=62, "XG_BIAS_LOW"=64, "XG_BIAS_HIGH"=66, "YG_BIAS_LOW"=68, "YG_BIAS_HIGH"=70, "ZG_BIAS_LOW"=72, "ZG_BIAS_HIGH"=74, "XA_BIAS_LOW"=76, "XA_BIAS_HIGH"=78, "YA_BIAS_LOW"=80, "YA_BIAS_HIGH"=82, "ZA_BIAS_LOW"=84, "ZA_BIAS_HIGH"=86, "Reserved5"=88, "Reserved6"=90, "FILT_CTRL"=92, "Reserved5"=94, "MSC_CTRL"=96, "UP_SCALE"=98, "DEC_RATE"=100, "NULL_CNFG"=102, "GLOB_CMD"=104, "Reserved6"=106, "FIRM_REV"=108, "FIRM_DM"=110, "FIRM_Y"=112, "PROD_ID"=114, "SERIAL_NUM"=116, "USER_SCR1"=118, "USER_SCR2"=120, "USER_SCR3"=122, "FLSHCNT_LOW"=124, "FLSHCNT_HIGH"=126] ("Registers")
        # "Status LED on PCB wired to CS3 on Rio SPI Port"
        # "An extra two bytes are needed to complete the read. NULL bytes were added because the AutoSPI controller \nonly supports byte (8-bit) transactions. The IMU requires two bytes (16-bits) per CS."
        n77 = Unbundle By Name(w209) -> ("Data Ready Source"=w197:T13, "SPIDevRef.SPI Bus"=w196:T11, "ADIS16470DevRef.Hardware Config.Stall Config"=w200:T31, "DMARef"=w192:T20)
        n78 = call <vilib>:"FPGA_SPI_ConfigureAuto.vi"("SPI Auto Zero Byte Count"=u8 0, "error in"=w216, "SPI Auto TX Byte Array"=w198, "Stall Config"=w200, "SPI Bus"=w196) -> ("error out"=w214:errorcluster)  [unwired: 6 in]
        n79 = call <vilib>:"FPGA_SPI_StartAuto_External.vi"("error in (no error)"=w214, "Falling Edge"=FALSE, "Rising Edge"=TRUE, "Source"=w197) -> ("error out"=w210:errorcluster)  [unwired: 7 in]
        n80 = Array Size(array=w198) -> (size(s)=w207:i32)
        n81 = call <vilib>:"WPI_DigitalOutputOpen.vi"("error in (no error)"=w210, "DIO Channel"=FPGA_DIOChannel."SPI Port CS3") -> ("error out"=w206:errorcluster, "DigitalOutputDevRef"=w205:T27)  [unwired: 8 in]
        n82 = Bundle By Name(cluster=w209, "Bytes Per Sample"=w207, "Data Packet"=w198, "AutoSPI Active?"=TRUE) -> (w208:T21)
        n83 = call "Set Indicator LEDs.vi"("LED Index"=Indicator_LED_Indexes."Gyro Calibrated", "Color"=T25 1851904) -> ()  [unwired: 9 in, 1 out]
        n84 = call <vilib>:"WPI_DigitalOutputSetValue.vi"("error in (no error)"=w206, "Value"=FALSE, "DigitalOutputDevRef"=w205) -> ("error out"=w203:errorcluster, "DigitalOutputDevRef"=w202:T27)  [unwired: 7 in]
        n85 = call <vilib>:"WPI_DigitalOutputRefNum Registry Set.vi"("error in (no error)"=w203, "refnum name"="470 Status LED", "DigitalOutputDevRef"=w202) -> ("error out"=w194:errorcluster)  [unwired: 7 in, 1 out]
        n86 = call <vilib>:"WPI_DMAStart.vi"("error in (no error)"=w194, "DMARef"=w192) -> ("error out"=w193:errorcluster)  [unwired: 8 in, 1 out]
      }
      frame "Decode AutoSPI" {
        # "Main data capture and accumulation loop. Only active if AutoSPI is enabled."
        n87 = Unbundle By Name(w219) -> ("AutoSPI Active?"=w218:bool)
        n88 = case shown="True" w218 {
          tunnel: [w224 w242] -> w222
          tunnel: w221 -> [w223 w226]
          tunnel: [w223 w229] -> w220
          tunnel: w219 -> [w224 w233]
          tunnel: w219 -> [_ w231]
          frame False {
          }
          frame True {
            n89 = Unbundle By Name(w231) -> ("Reset"=w240:bool, "Data"=w238:dbl[], "Bytes Per Sample"=w239:u32)
            n90 = Unbundle By Name(w231) -> ("TimeStampPrev"=w230:u32)
            n91 = call "ADIS16470 Decode AutoSPI.vi"("error in (no error)"=w226, "TimeStampPrev"=w230, "Bytes Per Sample"=w239, "Data in"=w238) -> ("error out"=w229:errorcluster, "Last Timestamp"=w232:u32, "Data out"=w237:dbl[], "Raw Data"=w227:cluster{"Theta":dbl[], "Timestamp":u32}[])  [unwired: 4 in]
            n92 = call "Sample Encoder DMA.vi"("error in (no error)"=w226) -> ("Array"=w225:T32)  [unwired: 9 in, 1 out]
            n93 = Select(t=dbl[] [0.0, 0.0, 0.0, 0.0, 0.0, 0.0, 0.0, 0.0] ("Angle and Vel"), s=w240, f=w237) -> (s? t:f=w236:dbl[])
            n94 = Index Array(array=w236, index=3) -> (element=→"Waveform Chart":dbl)
            n95 = Bundle By Name(cluster=w233, "Reset"=FALSE ("First Run"), "Data"=w236, "TimeStampPrev"=w232, "IMU Raw"=w227, "Encoder Raw"=w225) -> (w242:T21)
          }
        }
      }
      frame "Process" {
        n96 = disable-structure shown="Disabled" {
          disable-tunnel: w247 -> [w259 _ w273]
          disable-tunnel: w246 -> [w257 _ w274]
          disable-tunnel: [w256 _ w274] -> w245
          frame Disabled {
            n97 = Unbundle By Name(w259) -> ("ADIS16470DevRef.Sychronous Process VI"=w254:T12, "ADIS16470DevRef.Data FIFO"=w258:refnum<k33>, "Data"=w253:dbl[])
            n98 = Index Array(array=w253) -> (element #1=w252:dbl, element #2=w251:dbl, element #3=w250:dbl)  [unwired: 3 in]
            n99 = Bundle By Name(cluster="element", "XAngle"=w252, "YAngle"=w251, "ZAngle"=w250) -> (w248:T6)
            n100 = RT FIFO Write(0:w258, 1:w248) -> ()  [unwired: 3 in, 4 out]
            n101 = Not A Number/Path/Refnum?(number/path/refnum=w254) -> (NaN/Path/Refnum?=w255:bool)
            n102 = case shown="True" w255 {
              tunnel: w257 -> [w260 w265]
              tunnel: w248 -> [_ _]
              tunnel: [w264 w265] -> w256
              tunnel: w254 -> [w263 _]
              frame False {
                n103 = call-by-ref "?"(reference=w263, error in=w260, 8:"error in (no error)"=w260) -> (error out=w261:errorcluster, 0:"error out"=w262:errorcluster)  [unwired: 10 in, 1 out]
                n104 = Merge Errors(w261, w262) -> (w264:errorcluster)
              }
              frame True {
              }
            }
          }
          frame Enabled {
          }
          frame Disabled {
            n105 = Unbundle By Name(w273) -> ("IMU Raw"=w272:cluster{"Theta":dbl[], "Timestamp":u32}[], "Encoder Raw"=w271:T33)
            n106 = for {
              tunnel: w272 -> [w281] mode=indexing
              tunnel: [w280] -> _ mode=indexing
              tunnel: [w279] -> w270 mode=indexing
              n107 = Unbundle By Name(w281) -> ("Theta"=w280:dbl[], "Timestamp"=w279:u32)
            }
            "Array" <- w270
            n108 = for {
              tunnel: w271 -> [w278] mode=indexing
              tunnel: [w277] -> w268 mode=indexing
              tunnel: [w276] -> _ mode=indexing
              tunnel: [w275] -> _ mode=indexing
              n109 = Unbundle By Name(w278) -> ("Encoder R"=w275:u32, "Encoder L"=w276:u32, "Timestamp"=w277:u32)
            }
            "Array 2" <- w268
            n110 = feedback-in #1(w270) -> ()
            n111 = feedback #1() -> (→"ArrayPrev":u32[])  [unwired: 1 in]
            n112 = feedback #2() -> (→"Array2Prev":u32[])  [unwired: 1 in]
            n113 = feedback-in #2(w268) -> ()
            n114 = Wait (ms)(milliseconds to wait=u32 10) -> ()  [unwired: 1 out]
          }
        }
      }
      frame "Run Cmds" {
        n115 = Unbundle By Name(w284) -> ("ADIS16470DevRef.Cmd FIFO"=w294:refnum<k33>)
        n116 = Unbundle By Name(w284) -> ("SPIDevRef"=w283:T18, "ADIS16470DevRef.Status FIFO"=w289:refnum<k33>, "ADIS16470DevRef.Calibration Complete"=w290:refnum<notifier>)
        n117 = RT FIFO Read(0:w294, 1:T26 {"Command"=enum."None", "Data"=0} ("element")) -> (8:w288:refnum<k33>, 9:w287:T26)  [unwired: 2 in, 3 out]
        n118 = Unbundle By Name(w287) -> ("Command"=w286:T34, "Data"=w285:u32)
        n119 = case shown="\"Recal Complete\"" w286 {
          tunnel: w284 -> [w296 w301 w309 w314 w328 w337 w382]
          tunnel: w293 -> [w297 w300 w304 w312 w333 w360 w392]
          tunnel: [w297 w300 w303 w311 w333 w343 w380] -> w292
          tunnel: [w296 w299 w309 w315 w327 w336 w382] -> w291
          tunnel: w290 -> [_ _ _ _ w332 _ _]
          tunnel: w289 -> [_ _ _ w319 w330 _ _]
          tunnel: w288 -> [_ _ _ w317 _ w358 w394]
          tunnel: w285 -> [_ _ w305 _ _ _ _]
          tunnel: w284 -> [_ _ _ _ _ w357 w385]
          tunnel: w283 -> [_ _ w302 w310 _ w334 _]
          frame "None", Default {
          }
          frame "Reset" {
            n120 = Bundle By Name(cluster=w301, "Reset"=TRUE ("First Run")) -> (w299:T21)
          }
          frame "Set Calibration Period" {
            w307 = T19 102 items=["Reserved1"=0, "DIAG_STAT"=2, "X_GYRO_LOW"=4, "X_GYRO_OUT"=6, "Y_GYRO_LOW"=8, "Y_GYRO_OUT"=10, "Z_GYRO_LOW"=12, "Z_GYRO_OUT"=14, "X_ACCL_LOW"=16, "X_ACCL_OUT"=18, "Y_ACCL_LOW"=20, "Y_ACCL_OUT"=22, "Z_ACCL_LOW"=24, "Z_ACCL_OUT"=26, "TEMP_OUT"=28, "TIME_STAMP"=30, "Reseved2"=32, "DATA_CNTR"=34, "X_DELTANG_LOW"=36, "X_DELTANG_OUT"=38, "Y_DELTANG_LOW"=40, "Y_DELTANG_OUT"=42, "Z_DELTANG_LOW"=44, "Z_DELTANG_OUT"=46, "X_DELTVEL_LOW"=48, "X_DELTVEL_OUT"=50, "Y_DELTVEL_LOW"=52, "Y_DELTVEL_OUT"=54, "Z_DELTVEL_LOW"=56, "Z_DELTVEL_OUT"=58, "Reserved3"=60, "Reserved4"=62, "XG_BIAS_LOW"=64, "XG_BIAS_HIGH"=66, "YG_BIAS_LOW"=68, "YG_BIAS_OUT"=70, "ZG_BIAS_LOW"=72, "ZG_BIAS_OUT"=74, "XA_BIAS_LOW"=76, "XA_BIAS_HIGH"=78, "YA_BIAS_LOW"=80, "YA_BIAS_OUT"=82, "ZA_BIAS_LOW"=84, "ZA_BIAS_OUT"=86, "Reserved5"=88, "Reserved6"=90, "FILT_CTRL"=92, "Reserved5"=94, "MSC_CTRL"=96, "UP_SCALE"=98, "DEC_RATE"=100, "NULL_CNFG"=102, "GLOB_CMD"=104, "Reserved6"=106, "FIRM_REV"=108, "FIRM_DM"=110, "FIRM_Y"=112, "PROD_ID"=114, "SERIAL_NUM"=116, "USER_SCR1"=118, "USER_SCR2"=120, "USER_SCR3"=122, "FLSHCNT_LOW"=124, "FLSHCNT_HIGH"=126] ("Register")
            w308 = 1792  # Data
            n121 = Or(x=w305, y=w308) -> (x .or. y?=w306:u32)
            n122 = call "ADIS16470 Write Register.vi"("error in (no error)"=w304, "Data"=w306, "Register"=w307, "SPIDevRef in"=w302) -> ("error out"=w303:errorcluster)  [unwired: 6 in, 1 out]
          }
          frame "Recalibrate" {
            w320 = T19 104 items=["Reserved1"=0, "DIAG_STAT"=2, "X_GYRO_LOW"=4, "X_GYRO_OUT"=6, "Y_GYRO_LOW"=8, "Y_GYRO_OUT"=10, "Z_GYRO_LOW"=12, "Z_GYRO_OUT"=14, "X_ACCL_LOW"=16, "X_ACCL_OUT"=18, "Y_ACCL_LOW"=20, "Y_ACCL_OUT"=22, "Z_ACCL_LOW"=24, "Z_ACCL_OUT"=26, "TEMP_OUT"=28, "TIME_STAMP"=30, "Reseved2"=32, "DATA_CNTR"=34, "X_DELTANG_LOW"=36, "X_DELTANG_OUT"=38, "Y_DELTANG_LOW"=40, "Y_DELTANG_OUT"=42, "Z_DELTANG_LOW"=44, "Z_DELTANG_OUT"=46, "X_DELTVEL_LOW"=48, "X_DELTVEL_OUT"=50, "Y_DELTVEL_LOW"=52, "Y_DELTVEL_OUT"=54, "Z_DELTVEL_LOW"=56, "Z_DELTVEL_OUT"=58, "Reserved3"=60, "Reserved4"=62, "XG_BIAS_LOW"=64, "XG_BIAS_HIGH"=66, "YG_BIAS_LOW"=68, "YG_BIAS_OUT"=70, "ZG_BIAS_LOW"=72, "ZG_BIAS_OUT"=74, "XA_BIAS_LOW"=76, "XA_BIAS_HIGH"=78, "YA_BIAS_LOW"=80, "YA_BIAS_OUT"=82, "ZA_BIAS_LOW"=84, "ZA_BIAS_OUT"=86, "Reserved5"=88, "Reserved6"=90, "FILT_CTRL"=92, "Reserved5"=94, "MSC_CTRL"=96, "UP_SCALE"=98, "DEC_RATE"=100, "NULL_CNFG"=102, "GLOB_CMD"=104, "Reserved6"=106, "FIRM_REV"=108, "FIRM_DM"=110, "FIRM_Y"=112, "PROD_ID"=114, "SERIAL_NUM"=116, "USER_SCR1"=118, "USER_SCR2"=120, "USER_SCR3"=122, "FLSHCNT_LOW"=124, "FLSHCNT_HIGH"=126] ("Register")
            w323 = u16 1  # Data
            # "Write Calibration"
            # "GLOB_CMD Timing"
            n123 = RT FIFO Write(0:w319, 1:T22 {"Calibrated?"=FALSE, "IMU Detected?"=TRUE} ("element")) -> ()  [unwired: 3 in, 4 out]
            n124 = RT FIFO Write(0:w317, 1:T26 {"Command"=enum."Start Auto SPI", "Data"=0} ("element")) -> ()  [unwired: 3 in, 4 out]
            n125 = call "ADIS16470 Write Register.vi"("error in (no error)"=w312, "Data"=w323, "Register"=w320, "SPIDevRef in"=w310) -> ("error out"=w322:errorcluster, "SPIDevRef out"=w321:T18)  [unwired: 6 in]
            n126 = flat-sequence {
              tunnel: w322 -> [w325]
              tunnel: [w325] -> w311
              tunnel: w321 -> [_]
              frame #0 {
                n127 = Wait (ms)(milliseconds to wait=u32 50) -> ()  [unwired: 1 out]
              }
            }
            n128 = Bundle By Name(cluster=w314, "Reset"=TRUE) -> (w315:T21)
          }
          frame "Recal Complete" {
            n129 = Send Notification(notification="", notifier=w332) -> ()  [unwired: 1 in, 2 out]
            n130 = RT FIFO Write(0:w330, 1:T22 {"Calibrated?"=TRUE, "IMU Detected?"=TRUE} ("element")) -> ()  [unwired: 3 in, 4 out]
            n131 = Bundle By Name(cluster=w328, "AutoSPI Active?"=TRUE) -> (w327:T21)
          }
          frame "Exit Auto SPI" {
            w353 = T19 114 items=["Reserved1"=0, "DIAG_STAT"=2, "X_GYRO_LOW"=4, "X_GYRO_OUT"=6, "Y_GYRO_LOW"=8, "Y_GYRO_OUT"=10, "Z_GYRO_LOW"=12, "Z_GYRO_OUT"=14, "X_ACCL_LOW"=16, "X_ACCL_OUT"=18, "Y_ACCL_LOW"=20, "Y_ACCL_OUT"=22, "Z_ACCL_LOW"=24, "Z_ACCL_OUT"=26, "TEMP_OUT"=28, "TIME_STAMP"=30, "Reseved2"=32, "DATA_CNTR"=34, "X_DELTANG_LOW"=36, "X_DELTANG_OUT"=38, "Y_DELTANG_LOW"=40, "Y_DELTANG_OUT"=42, "Z_DELTANG_LOW"=44, "Z_DELTANG_OUT"=46, "X_DELTVEL_LOW"=48, "X_DELTVEL_OUT"=50, "Y_DELTVEL_LOW"=52, "Y_DELTVEL_OUT"=54, "Z_DELTVEL_LOW"=56, "Z_DELTVEL_OUT"=58, "Reserved3"=60, "Reserved4"=62, "XG_BIAS_LOW"=64, "XG_BIAS_HIGH"=66, "YG_BIAS_LOW"=68, "YG_BIAS_OUT"=70, "ZG_BIAS_LOW"=72, "ZG_BIAS_OUT"=74, "XA_BIAS_LOW"=76, "XA_BIAS_HIGH"=78, "YA_BIAS_LOW"=80, "YA_BIAS_OUT"=82, "ZA_BIAS_LOW"=84, "ZA_BIAS_OUT"=86, "Reserved5"=88, "Reserved6"=90, "FILT_CTRL"=92, "Reserved5"=94, "MSC_CTRL"=96, "UP_SCALE"=98, "DEC_RATE"=100, "NULL_CNFG"=102, "GLOB_CMD"=104, "Reserved6"=106, "FIRM_REV"=108, "FIRM_DM"=110, "FIRM_Y"=112, "PROD_ID"=114, "SERIAL_NUM"=116, "USER_SCR1"=118, "USER_SCR2"=120, "USER_SCR3"=122, "FLSHCNT_LOW"=124, "FLSHCNT_HIGH"=126] ("ADIS16448 Register")
            n132 = Unbundle By Name(w357) -> ("ADIS16470DevRef.Hardware Config.IMU SPI Bus"=w356:T11, "ADIS16470DevRef.Hardware Config.SPI Clock Rate (Hz)"=w355:dbl, "ADIS16470DevRef.Hardware Config.IMU SPI Mode (3)"=w354:T9)
            n133 = call <vilib>:"WPI_SPIClose.vi"("error in (no error)"=w360, "SPIDevRef"=w334) -> ("error out"=w339:errorcluster)  [unwired: 9 in]
            n134 = call <vilib>:"WPI_DigitalOutputRefNum Registry Get.vi"("error in (no error)"=w339, "refnum name"="470 Status LED") -> ("error out"=w341:errorcluster, "DigitalOutputDevRef"=w340:T27)  [unwired: 8 in]
            n135 = call <vilib>:"WPI_DigitalOutputSetValue.vi"("error in (no error)"=w341, "Value"=TRUE, "DigitalOutputDevRef"=w340) -> ("error out"=w338:errorcluster)  [unwired: 7 in, 1 out]
            n136 = RT FIFO Write(0:w358, 1:T26 {"Command"=enum."Recalibrate", "Data"=0} ("element")) -> ()  [unwired: 3 in, 4 out]
            n137 = call <vilib>:"WPI_SPIOpen.vi"("error in"=w338, "Mode (3)"=w354, "Clock Rate (Hz)"=w355, "SPI Bus"=w356) -> ("error out"=w352:errorcluster, "SPIDevRef"=w345:T18)  [unwired: 6 in]
            n138 = call "ADIS16470 Read Register.vi"("error in (no error)"=w352, "ADIS16470 Register"=w353, "SPIDevRef in"=w345) -> ("error out"=w346:errorcluster, "Register Value"=w344:u16, "SPIDevRef out"=w347:T18)  [unwired: 6 in]
            n139 = Or(x=u16 16982 ("y"), y=u16 16470) -> (x .or. y?=w349:u16)
            n140 = Equal?(x=w349, y=w344) -> (x = y?=w348:bool)
            n141 = case shown="True" w348 {
              tunnel: w347 -> [_ w374]
              tunnel: w346 -> [w363 w373]
              tunnel: [w362 w372] -> w343
              tunnel: w337 -> [w361 w370]
              tunnel: [w361 w369] -> w336
              frame False {
                n142 = case shown="No Error" w363 {
                  selector: w363 -> [w365 w368]
                  tunnel: [w364 w368] -> w362
                  frame No Error {
                    n143 = call <vilib>:"Error Cluster From Error Code.vi"("error in (no error)"=w365, "error message (\"\")"="SPI port did not reset properly" ("error message (\"\")"), "error code (0)"=-8106) -> ("error out"=w364:errorcluster)  [unwired: 6 in]
                  }
                  frame Error {
                  }
                }
              }
              frame True {
                n144 = call <vilib>:"WPI_SPIRefNum Registry Set.vi"("error in (no error)"=w373, "refnum name"="AutoSPI", "SPIDevRef"=w374) -> ("error out"=w372:errorcluster, "SPIDevRef"=w375:T18)  [unwired: 7 in]
                n145 = Bundle By Name(cluster=w370, "SPIDevRef"=w375, "AutoSPI Active?"=FALSE) -> (w369:T21)
              }
            }
          }
          frame "Start Auto SPI" {
            n146 = Unbundle By Name(w385) -> ("Data Ready Source"=w384:T13, "SPIDevRef.SPI Bus"=w379:T11, "ADIS16470DevRef.Hardware Config.Stall Config"=w378:T31, "Data Packet"=w377:T19[])
            n147 = RT FIFO Write(0:w394, 1:T26 {"Command"=enum."Recal Complete", "Data"=0} ("element")) -> ()  [unwired: 3 in, 4 out]
            n148 = call <vilib>:"FPGA_SPI_ConfigureAuto.vi"("SPI Auto Zero Byte Count"=u8 0, "error in"=w392, "SPI Auto TX Byte Array"=w377, "Stall Config"=w378, "SPI Bus"=w379) -> ("error out"=w383:errorcluster)  [unwired: 6 in]
            n149 = call <vilib>:"FPGA_SPI_StartAuto_External.vi"("error in (no error)"=w383, "Falling Edge"=TRUE, "Rising Edge"=FALSE, "Source"=w384) -> ("error out"=w389:errorcluster)  [unwired: 7 in]
            n150 = call <vilib>:"WPI_DigitalOutputRefNum Registry Get.vi"("error in (no error)"=w389, "refnum name"="470 Status LED") -> ("error out"=w388:errorcluster, "DigitalOutputDevRef"=w387:T27)  [unwired: 8 in]
            n151 = call <vilib>:"WPI_DigitalOutputSetValue.vi"("error in (no error)"=w388, "Value"=FALSE, "DigitalOutputDevRef"=w387) -> ("error out"=w380:errorcluster)  [unwired: 7 in, 1 out]
          }
        }
      }
      frame "Close" {
        n152 = call <vilib>:"WPI_DigitalOutputRefNum Registry Get.vi"("refnum name"="470 Status LED") -> ("error out"=w407:errorcluster, "DigitalOutputDevRef"=w406:T27)  [unwired: 9 in]
        n153 = call <vilib>:"WPI_DigitalOutputClose.vi"("error in (no error)"=w407, "DigitalOutputDevRef"=w406) -> ("error out"=w405:errorcluster)  [unwired: 9 in]
        n154 = call <vilib>:"WPI_DigitalOutputRefNum Registry Get.vi"("error in (no error)"=w405, "refnum name"="470 Reset Pin") -> ("error out"=w403:errorcluster, "DigitalOutputDevRef"=w402:T27)  [unwired: 8 in]
        n155 = call <vilib>:"WPI_DigitalOutputClose.vi"("error in (no error)"=w403, "DigitalOutputDevRef"=w402) -> ("error out"=w401:errorcluster)  [unwired: 9 in]
        n156 = call <vilib>:"WPI_SPIRefNum Registry Get.vi"("error in (no error)"=w401, "refnum name"="AutoSPI") -> ("error out"=w399:errorcluster, "SPIDevRef"=w398:T18)  [unwired: 8 in]
        n157 = call <vilib>:"WPI_SPIClose.vi"("error in (no error)"=w399, "SPIDevRef"=w398) -> ()  [unwired: 9 in, 1 out]
      }
    }
  }
  "error out" <- w1
